vi "全局变量.vi"() -> ()   [LabVIEW 2016, in "数据查询.lvlib"]
panel:
  in  "选择界面":T1=enum."仪器数据"
  in  "数据库类型":enum16{"Access", "SQLite"}(ring)
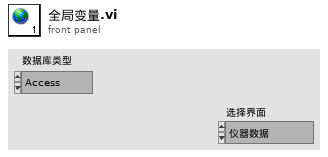
[diagram p1: front panel]
types:
  T1 = typedef "数据查询菜单.xctl/数据 1.ctl" = enum32{"数据查询", "仪器数据", "仪器日志", "报警信息", "校准日志"}
diagram:
